vi "configureGlobal.vi"(8 "error in (no error)":errorcluster, 10 "Data":u8[](array[numeric]), 11 "Mockbus in":refnum<class "Mockbus.lvclass">) -> (0 "error out":errorcluster, 3 "Mockbus out":refnum<class "Mockbus.lvclass">)   [LabVIEW 2015, in "RTMockbus.lvlib" / "Mockbus.lvclass"]
uses:
  Mockbus.lvclass
  Mockbus.lvclass/Mockbus.ctl
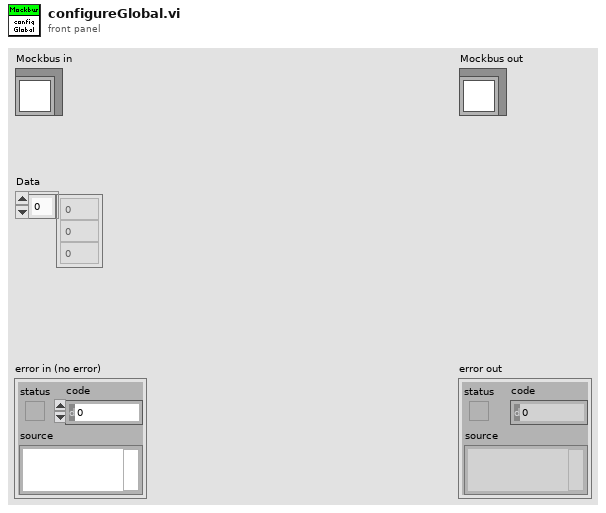
[diagram p1: front panel]
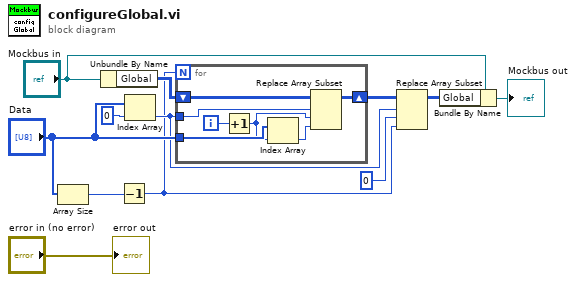
[diagram p0: block diagram]
diagram:
  n1 = Array Size(array="Data") -> (size(s)=w10:i32)
  n2 = Unbundle By Name("Mockbus in") -> ("Global"=w11:u8[][])
  n3 = Decrement(x=w10) -> (x-1=w5:i32)
  n4 = Index Array(array="Data", index=0) -> (element=w6:u8)
  n5 = for {
    N: w5 -> [_]
    tunnel: w6 -> [w16]
    tunnel: "Data" -> [w18]
    shift-right: [w13] -> w8
    shift-left: w11 -> [w17]
    i -> [w19]
    n6 = Increment(x=w19) -> (x+1=w15:i32)
    n7 = Index Array(array=w18, index=w15) -> (element=w14:u8)
    n8 = Replace Array Subset(array=w17, new element=w14, index (row)=w16, index (col)=w15) -> (w13:u8[][])
  }
  n9 = Replace Array Subset(array=w8, new element=w5, index (row)=w6, index (col)=0 ("index (row)")) -> (w3:u8[][])
  n10 = Bundle By Name(cluster="Mockbus in", "Global"=w3) -> (→"Mockbus out":refnum<class "Mockbus.lvclass">)
  "error out" <- "error in (no error)"
